vi "wave 2.vi"() -> ()   [LabVIEW 2011]
panel:
  out "Waveform Chart 2":dbl(graph)
  out "Waveform Chart":dbl(graph)
  in  "Numeric":dbl
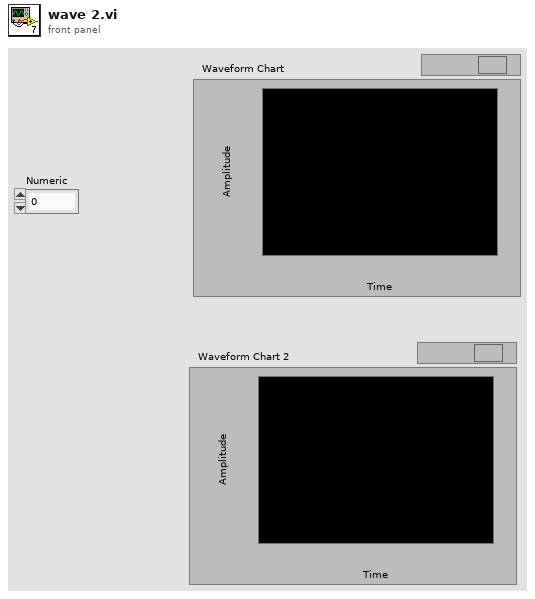
[diagram p1: front panel]
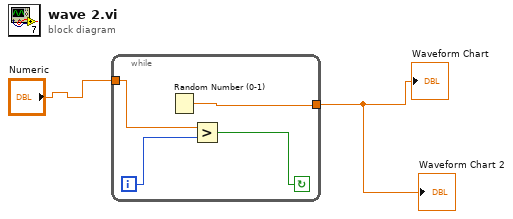
[diagram p0: block diagram]
diagram:
  n1 = while {
    tunnel: [w6] -> w2
    tunnel: "Numeric" -> [w5]
    i -> [w3]
    stop <- w4 continue-if-true
    n2 = Random Number (0-1)() -> (number: 0 to 1=w6:dbl)
    n3 = Greater?(x=w5, y=w3) -> (0:w4:bool)
  }
  "Waveform Chart" <- w2
  "Waveform Chart 2" <- w2
